vi "XIPIN_Binary_Counter_11_0.vi"   [LabVIEW 2017]
doc: "The Xilinx LogiCORE Binary Counter creates up counters, down counters, and up/down counters with output widths ranging up to 256 bits. The upper count limit is user programmable, and the counter's increment value can either be user-defined, or specified via an external input port.\n------------------------------------\n<b>Need License</b> : No"
uses:
  <vilib>/rvi/XilinxIP/XIPIN_XNode/niFpgaXIPIN.xnode
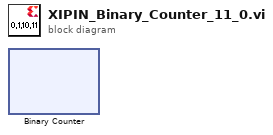
[diagram p0: block diagram]
diagram:
  n1 = xnode ("Binary Counter")() -> ()
